vi "Results_Row_Per_Channel.vi"(0 "Analysis_info_cluster":T1={"Colour"=0, "Inst type"=enum."Pitot-static tube", "Inst name"="Manometer voltage", "Symbol"="U", "Code name"="", "Extra Info"="U", "Inst Array"=enum."PWA", "Extra Titles"=[], "Extra Values"=[], "U"=0.0, "u^2"=0.0, "u^3"=0.0, "u^4"=0.0, "Skew_u"=0.0, "Kurt_u"=0.0, "Sd Error in Mean"=0.0, "% u'/U"=0.0, "X"=0.0, "Y"=0.0, "Z"=0.0, "Timescale integral to 25%"=0.0, "Sd Error in Variance"=0.0, "Calib File"=path "", "Calib Constants"=[], "Output Position"=FALSE, "Full Stats"=FALSE, "Av Sampling Rate"=0.0, "Av No of Samples"=0.0, "Total Meas Time (s)"=0.0, "ADAM Ch Name"=""} {"Sd Error in Variance" format="%.2f"; "Skew_u" format="%.2f"; "% u'/U" format="%.2f"; "Sd Error in Mean" format="%.2f"; "Kurt_u" format="%.2f"; "u^4" format="%.2f"; "u^3" format="%.2f"; "U" format="%.2f"; "u^2" format="%.2f"}) -> (1 "Channel Names":string[](array[string]), 2 "Channel Values":string[](array[string]))   [LabVIEW 2015]
uses:
  Controls/Analysis_info_cluster.ctl
  Controls/Inst_type.ctl
  Controls/Instrument_Array.ctl
  Controls/Post_Process.ctl
  Globals/Trav_pos_global.vi
  Acquisition/PWA/PWAtasksGLOBAL.vi
  Globals/Meas_global.vi
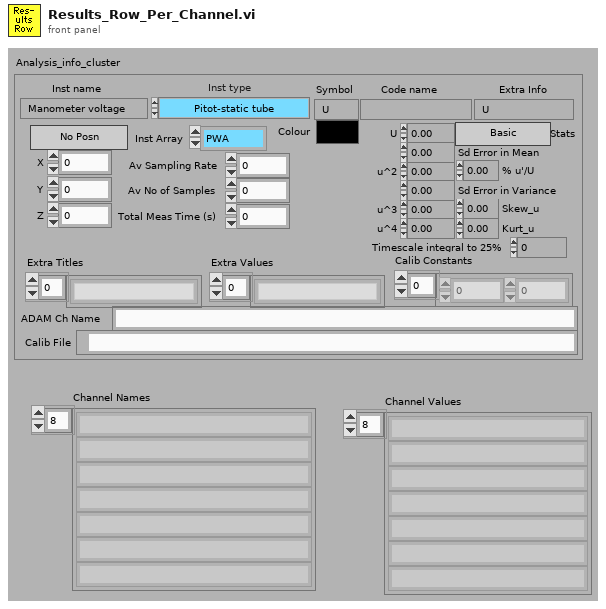
[diagram p1: front panel]
types:
  T1 = typedef "Analysis_info_cluster.ctl" = cluster{"Colour":u32, "Inst type":T2, "Inst name":string, "Symbol":string, "Code name":string, "Extra Info":string, "Inst Array":T3, "Extra Titles":string[], "Extra Values":string[], "U":dbl, "u^2":dbl, "u^3":dbl, "u^4":dbl, "Skew_u":dbl, "Kurt_u":dbl, "Sd Error in Mean":dbl, "% u'/U":dbl, "X":dbl, "Y":dbl, "Z":dbl, "Timescale integral to 25%":dbl, "Sd Error in Variance":dbl, "Calib File":path, "Calib Constants":dbl[], "Output Position":bool, "Full Stats":bool, "Av Sampling Rate":dbl, "Av No of Samples":dbl, "Total Meas Time (s)":dbl, "ADAM Ch Name":string}
  T2 = typedef "Inst_type.ctl" = enum16{"Propeller anemometer", "Raw voltage", "Pressure Transducer", "Pitot-static tube", "Preston tube", "Hot wire", "Cross wire 1", "Cross wire 2", "Generic Linear", "Generic Polynomial", "Generic BackPoly", "Fast FID", "Thermocouple", "Cold wire", "Pulsed Wire", "LDA Vel", "LDA Tran time", "LDA Arr time", "Microphone"}
  T3 = typedef "Instrument_Array.ctl" = enum16{"PWA", "LDA", "Analogue"}
  T4 = enum16{"Mean only", "2nd Order Stats", "4th Order Stats"}
  T5 = typedef "Post_Process.ctl" = enum16{"Take New Data", "Post Process Raw Data File"}
  T6 = typedef "Tunnel_Coordinates.ctl" = enum16{"Work in Tunnel Coordinates", "Work in Model Coordinates"}
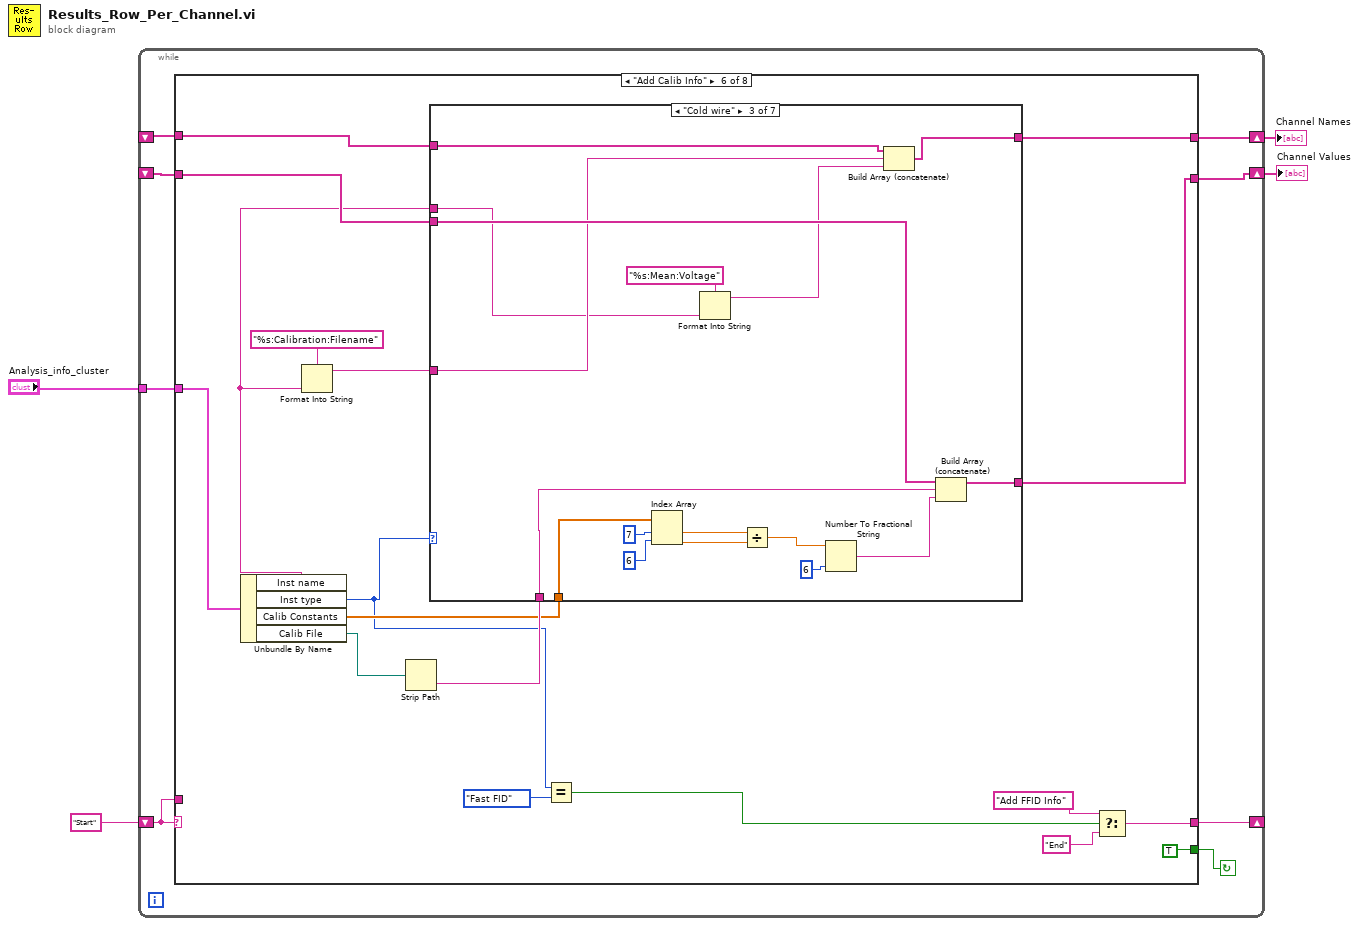
[diagram p0: block diagram]
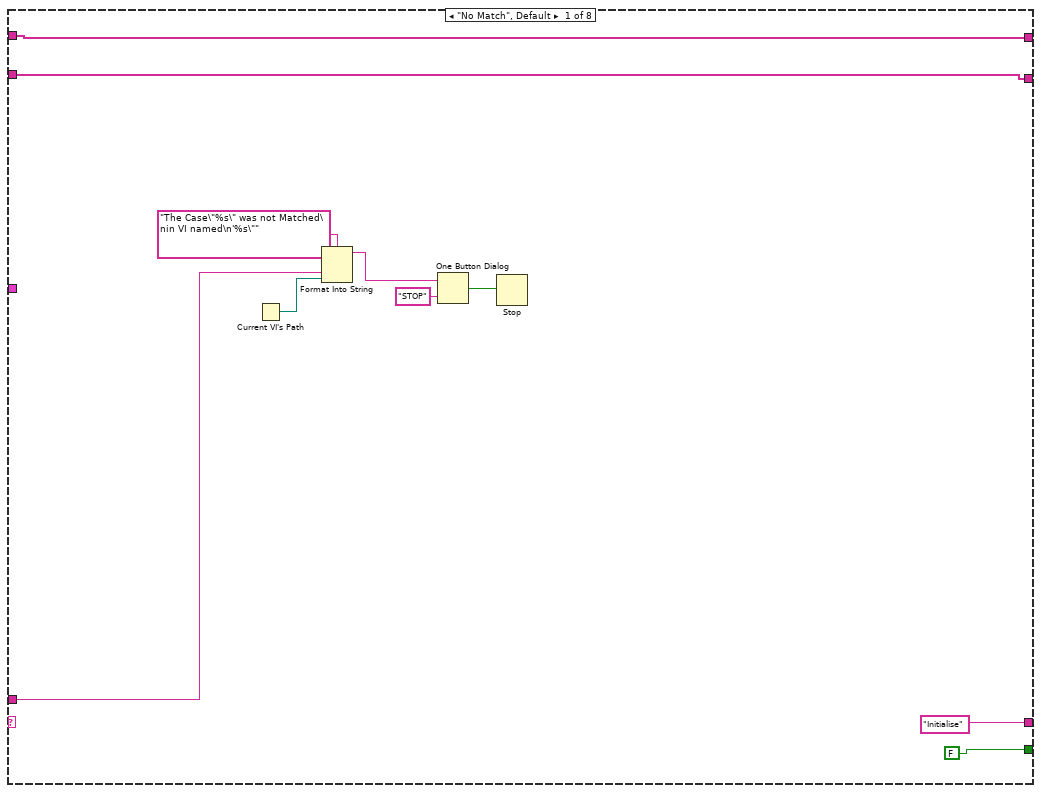
[diagram p2: hidden frame]
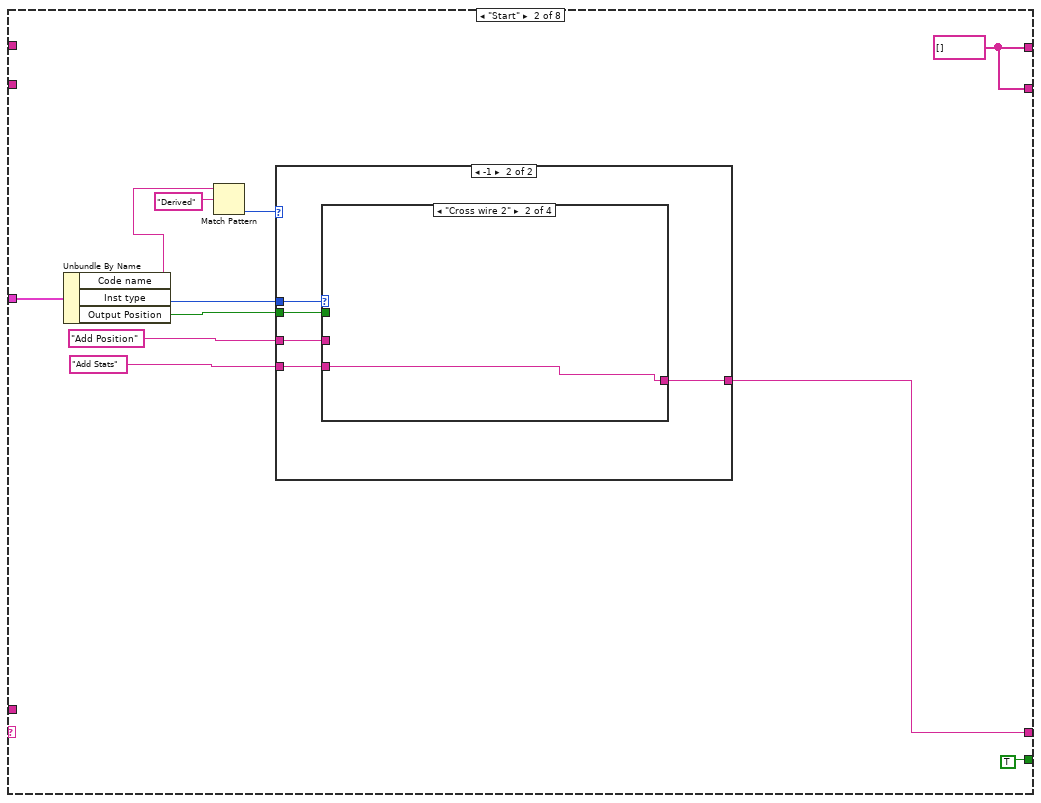
[diagram p3: hidden frame]
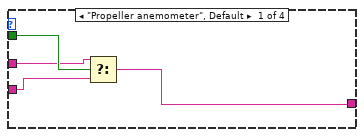
[diagram p5: hidden frame]
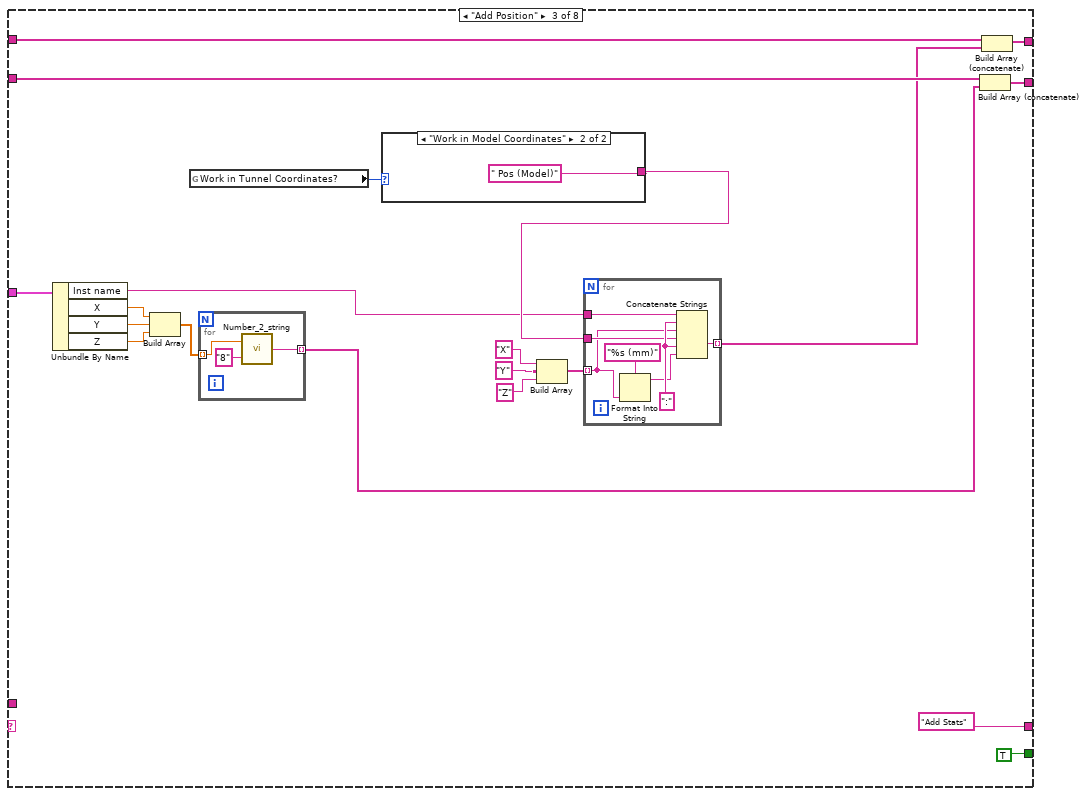
[diagram p8: hidden frame]
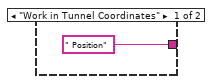
[diagram p9: hidden frame]
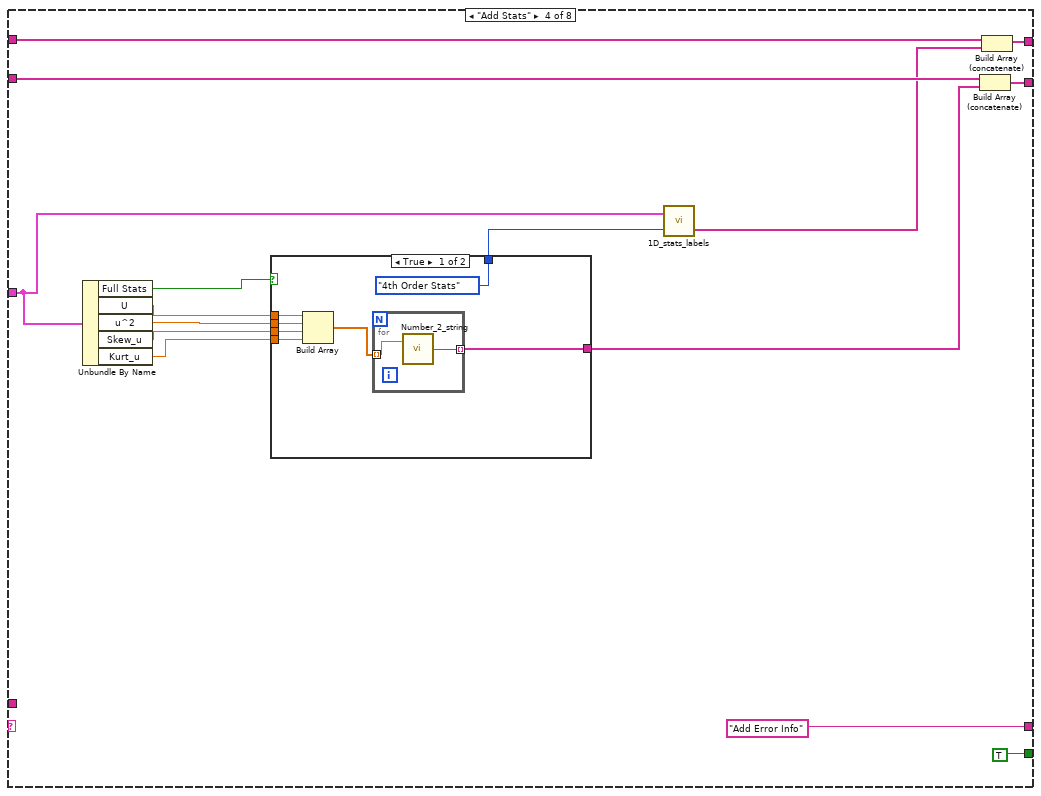
[diagram p10: hidden frame]
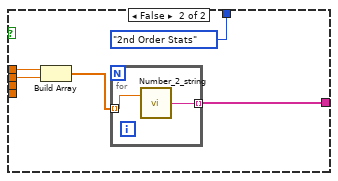
[diagram p11: hidden frame]
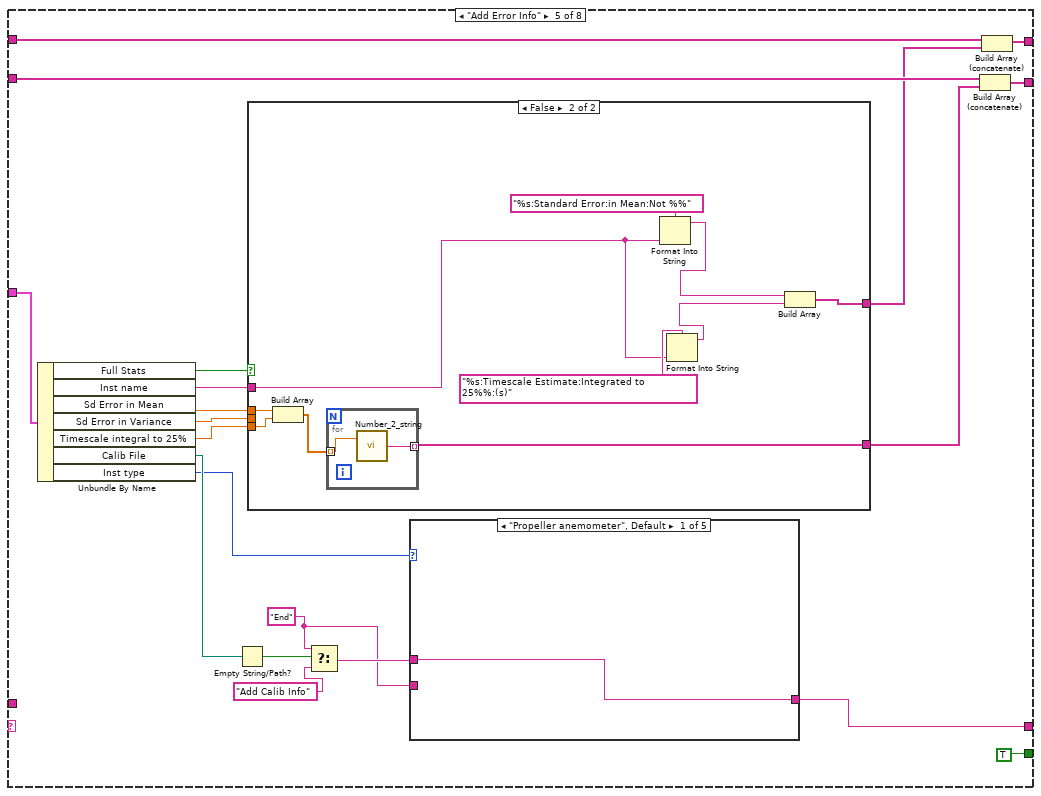
[diagram p12: hidden frame]
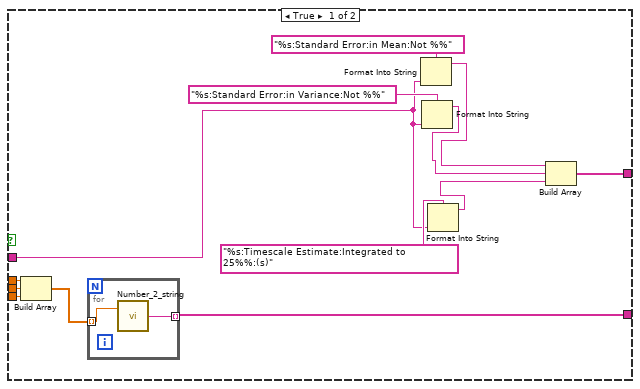
[diagram p13: hidden frame]
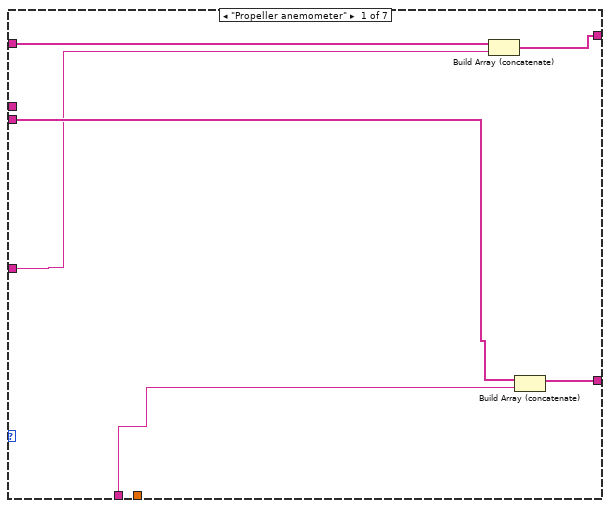
[diagram p18: hidden frame]
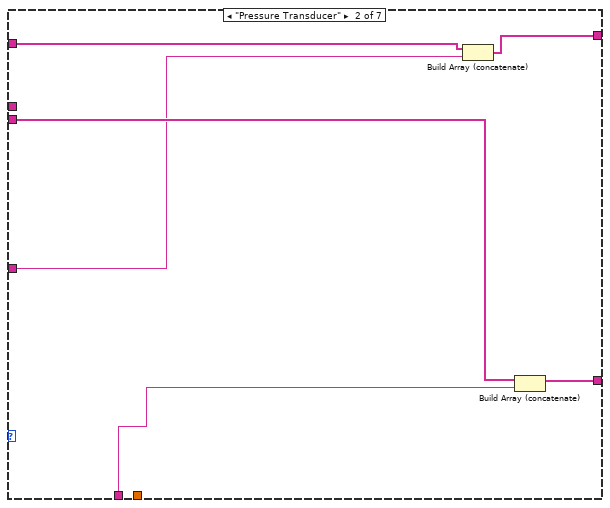
[diagram p19: hidden frame]
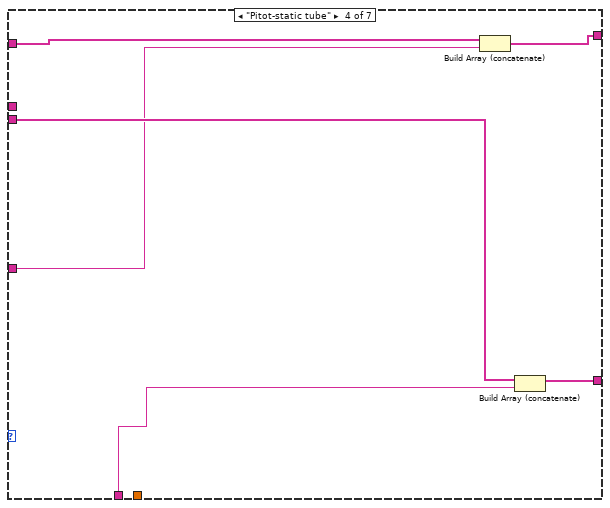
[diagram p20: hidden frame]
diagram:
  n1 = while {
    shift-left: "Start" -> [w10]
    shift-right: [w11] -> _
    shift-right: [w5] -> w1
    shift-left: _ -> [w6]
    shift-right: [w8] -> w2
    shift-left: _ -> [w7]
    tunnel: "Analysis_info_cluster" -> [w9]
    stop <- w12 continue-if-true
    n2 = case shown="\"Add Calib Info\"" w10 {
      tunnel: [FALSE TRUE TRUE TRUE TRUE TRUE TRUE FALSE] -> w12
      tunnel: ["Initialise" w30 "Add Stats" "Add Error Info" w113 w164 "End" "End"] -> w11
      tunnel: w10 -> [w18 _ _ _ _ _ _ _]
      tunnel: w9 -> [_ w32 w58 w84 w122 w178 w277 w298]
      tunnel: [w13 w28 w51 w89 w126 w174 w281 w292] -> w8
      tunnel: w7 -> [w13 _ w50 w88 w125 w176 w280 w295]
      tunnel: w6 -> [w14 _ w49 w87 w124 w171 w279 w297]
      tunnel: [w14 w28 w48 w86 w123 w169 w278 w293] -> w5
      frame "No Match", Default {
        n3 = Current VI's Path() -> (path=w17:path)
        n4 = Format Into String(format string="The Case\"%s\" was not Matched\nin VI named\n'%s\"" ("Format String"), w18, w17) -> (resulting string=w21:string)  [unwired: 2 in, 1 out]
        n5 = One Button Dialog(message=w21, button name ("OK")="STOP") -> (true=w19:bool)
        n6 = Stop(stop? (T)=w19) -> ()
      }
      frame "Start" {
        w28 = string[] []
        n7 = Unbundle By Name(w32) -> ("Code name"=w25:string, "Inst type"=w31:T2, "Output Position"=w23:bool)
        n8 = Match Pattern(string=w25, regular expression="Derived") -> (offset past match=w24:i32)  [unwired: 1 in, 3 out]
        n9 = case shown="-1" w24 {
          tunnel: w31 -> [_ w39]
          tunnel: [w34 w38] -> w30
          tunnel: "Add Position" -> [_ w37]
          tunnel: "Add Stats" -> [w34 w36]
          tunnel: w23 -> [_ w35]
          frame 0, Default {
          }
          frame -1 {
            n10 = case shown="\"Cross wire 2\"" w39 {
              tunnel: [w40 w44 w45 w46] -> w38
              tunnel: w37 -> [w42 _ _ _]
              tunnel: w36 -> [w41 w44 w45 w46]
              tunnel: w35 -> [w43 _ _ _]
              frame "Propeller anemometer", Default {
                n11 = Select(t=w42, s=w43, f=w41) -> (s? t:f=w40:string)
              }
              frame "Cross wire 2" {
              }
              frame "LDA Tran time" {
              }
              frame "LDA Arr time" {
              }
            }
          }
        }
      }
      frame "Add Position" {
        n12 = Unbundle By Name(w58) -> ("Inst name"=w57:string, "X"=w56:dbl, "Y"=w55:dbl, "Z"=w54:dbl)
        n13 = Build Array(w56, w55, w54) -> (w53:dbl[])
        n14 = global read "Trav_pos_global.vi" "Work in Tunnel Coordinates?"() -> (w64:T6)
        n15 = for {
          tunnel: w53 -> [w69] mode=indexing
          tunnel: [w68] -> w52 mode=indexing
          n16 = call "Number_2_string.vi"("precision"="8", "number"=w69) -> ("String"=w68:string)
        }
        n17 = case shown="\"Work in Model Coordinates\"" w64 {
          tunnel: [" Position" " Pos (Model)"] -> w59
          frame "Work in Tunnel Coordinates" {
          }
          frame "Work in Model Coordinates" {
          }
        }
        n18 = Build Array("X", "Y", "Z") -> (w63:string[])
        n19 = for {
          tunnel: w63 -> [w72] mode=indexing
          tunnel: w57 -> [w76]
          tunnel: [w74] -> w47 mode=indexing
          tunnel: w59 -> [w73]
          w75 = ":" ("Substring")
          n20 = Format Into String(format string="%s (mm)", w72) -> (resulting string=w70:string)  [unwired: 2 in, 1 out]
          n21 = Concatenate Strings(w76, w75, w72, w73, w75, w70) -> (w74:string)
        }
        n22 = Build Array (concatenate)(w50, w52) -> (w51:string[])
        n23 = Build Array (concatenate)(w49, w47) -> (w48:string[])
      }
      frame "Add Stats" {
        n24 = Unbundle By Name(w84) -> ("Full Stats"=w80:bool, "U"=w93:dbl, "u^2"=w92:dbl, "Skew_u"=w91:dbl, "Kurt_u"=w85:dbl)
        n25 = case shown="True" w80 {
          tunnel: w93 -> [w100 w107]
          tunnel: w92 -> [w99 w106]
          tunnel: w91 -> [w98 _]
          tunnel: [w96 w104] -> w90
          tunnel: w85 -> [w95 _]
          tunnel: [T4."4th Order Stats" ("Mode selector") T4."2nd Order Stats" ("Mode selector")] -> w81
          frame True {
            n26 = Build Array(w100, w99, w98, w95) -> (w97:dbl[])
            n27 = for {
              tunnel: w97 -> [w102] mode=indexing
              tunnel: [w101] -> w96 mode=indexing
              n28 = call "Number_2_string.vi"("number"=w102) -> ("String"=w101:string)  [unwired: 1 in]
            }
          }
          frame False {
            n29 = Build Array(w107, w106) -> (w105:dbl[])
            n30 = for {
              tunnel: w105 -> [w109] mode=indexing
              tunnel: [w108] -> w104 mode=indexing
              n31 = call "Number_2_string.vi"("number"=w109) -> ("String"=w108:string)  [unwired: 1 in]
            }
          }
        }
        n32 = call "1D_stats_labels.vi"("Mode selector"=w81, "Analysis Info Cluster"=w84) -> ("Output"=w83:string[])  [unwired: 1 in]
        n33 = Build Array (concatenate)(w88, w90) -> (w89:string[])
        n34 = Build Array (concatenate)(w87, w83) -> (w86:string[])
      }
      frame "Add Error Info" {
        w111 = "End"
        n35 = Unbundle By Name(w122) -> ("Full Stats"=w110:bool, "Inst name"=w121:string, "Sd Error in Mean"=w128:dbl, "Sd Error in Variance"=w119:dbl, "Timescale integral to 25%"=w118:dbl, "Calib File"=w117:path, "Inst type"=w112:T2)
        n36 = Empty String/Path?(string/path=w117) -> (empty?=w116:bool)
        n37 = case shown="False" w110 {
          tunnel: w128 -> [w142 w154]
          tunnel: [w140 w152] -> w127
          tunnel: w121 -> [w133 w147]
          tunnel: [w132 w146] -> w120
          tunnel: w119 -> [w131 _]
          tunnel: w118 -> [w130 w145]
          frame True {
            n38 = Build Array(w142, w131, w130) -> (w141:dbl[])
            n39 = for {
              tunnel: w141 -> [w144] mode=indexing
              tunnel: [w143] -> w140 mode=indexing
              n40 = call "Number_2_string.vi"("number"=w144) -> ("String"=w143:string)  [unwired: 1 in]
            }
            n41 = Format Into String(format string="%s:Standard Error:in Mean:Not %%", w133) -> (resulting string=w135:string)  [unwired: 2 in, 1 out]
            n42 = Format Into String(format string="%s:Standard Error:in Variance:Not %%", w133) -> (resulting string=w137:string)  [unwired: 2 in, 1 out]
            n43 = Format Into String(format string="%s:Timescale Estimate:Integrated to 25%%:(s)", w133) -> (resulting string=w139:string)  [unwired: 2 in, 1 out]
            n44 = Build Array(w135, w137, w139) -> (w132:string[])
          }
          frame False {
            n45 = Build Array(w154, w145) -> (w153:dbl[])
            n46 = for {
              tunnel: w153 -> [w156] mode=indexing
              tunnel: [w155] -> w152 mode=indexing
              n47 = call "Number_2_string.vi"("number"=w156) -> ("String"=w155:string)  [unwired: 1 in]
            }
            n48 = Format Into String(format string="%s:Standard Error:in Mean:Not %%", w147) -> (resulting string=w149:string)  [unwired: 2 in, 1 out]
            n49 = Format Into String(format string="%s:Timescale Estimate:Integrated to 25%%:(s)", w147) -> (resulting string=w151:string)  [unwired: 2 in, 1 out]
            n50 = Build Array(w149, w151) -> (w146:string[])
          }
        }
        n51 = Select(t=w111, s=w116, f="Add Calib Info") -> (s? t:f=w114:string)
        n52 = case shown="\"Propeller anemometer\", Default" w112 {
          tunnel: [w157 w158 w159 w160 w161] -> w113
          tunnel: w114 -> [w157 _ _ _ _]
          tunnel: w111 -> [_ w158 w159 w160 w161]
          frame "Propeller anemometer", Default {
          }
          frame "Cross wire 2" {
          }
          frame "LDA Tran time" {
          }
          frame "LDA Arr time" {
          }
          frame "Raw voltage" {
          }
        }
        n53 = Build Array (concatenate)(w125, w127) -> (w126:string[])
        n54 = Build Array (concatenate)(w124, w120) -> (w123:string[])
      }
      frame "Add Calib Info" {
        n55 = Unbundle By Name(w178) -> ("Inst name"=w168:string, "Inst type"=w167:T2, "Calib Constants"=w173:dbl[], "Calib File"=w177:path)
        n56 = Format Into String(format string="%s:Calibration:Filename" ("Format String"), w168) -> (resulting string=w170:string)  [unwired: 2 in, 1 out]
        n57 = Strip Path(path=w177) -> (name=w175:string)  [unwired: 1 out]
        n58 = case shown="\"Cold wire\"" w167 {
          tunnel: [w185 w190 w207 w213 w219 w226 w249] -> w174
          tunnel: w176 -> [w183 w191 w208 w214 w220 w227 w250]
          tunnel: w175 -> [w184 w189 w206 w212 w218 _ w243]
          tunnel: w173 -> [_ _ w199 _ _ _ w242]
          tunnel: w171 -> [w182 w188 w205 w211 w217 w223 w235]
          tunnel: w170 -> [w180 w187 w204 w209 w216 w221 w234]
          tunnel: [w181 w186 w203 w210 w215 w222 w229] -> w169
          tunnel: w168 -> [_ _ w201 _ _ _ w228]
          frame "Propeller anemometer" {
            n59 = Build Array (concatenate)(w182, w180) -> (w181:string[])
            n60 = Build Array (concatenate)(w183, w184) -> (w185:string[])
          }
          frame "Pressure Transducer" {
            n61 = Build Array (concatenate)(w188, w187) -> (w186:string[])
            n62 = Build Array (concatenate)(w191, w189) -> (w190:string[])
          }
          frame "Cold wire" {
            n63 = Index Array(array=w199, index #1=7 ("index"), index #2=6 ("index")) -> (element #1=w193:dbl, element #2=w192:dbl)
            n64 = Format Into String(format string="%s:Mean:Voltage" ("Format String"), w201) -> (resulting string=w200:string)  [unwired: 2 in, 1 out]
            n65 = Divide(x=w193, y=w192) -> (x/y=w197:dbl)
            n66 = Number To Fractional String(number=w197, precision (6)=i16 6) -> (F-format string=w195:string)  [unwired: 2 in]
            n67 = Build Array (concatenate)(w205, w204, w200) -> (w203:string[])
            n68 = Build Array (concatenate)(w208, w206, w195) -> (w207:string[])
          }
          frame "Pitot-static tube" {
            n69 = Build Array (concatenate)(w211, w209) -> (w210:string[])
            n70 = Build Array (concatenate)(w214, w212) -> (w213:string[])
          }
          frame "Preston tube" {
            n71 = Build Array (concatenate)(w220, w218) -> (w219:string[])
            n72 = Build Array (concatenate)(w217, w216) -> (w215:string[])
          }
          frame "Pulsed Wire" {
            n73 = global read "PWAtasksGLOBAL.vi" "PWA Calib. File Path"() -> (w225:path)
            n74 = Strip Path(path=w225) -> (name=w224:string)  [unwired: 1 out]
            n75 = Build Array (concatenate)(w223, w221) -> (w222:string[])
            n76 = Build Array (concatenate)(w227, w224) -> (w226:string[])
          }
          frame "Generic Linear", Default {
            n77 = global read "Meas_global.vi" "Post Process"() -> (w245:T5)
            n78 = Index Array(array=w242, index=18 ("Index")) -> (element=w248:dbl)
            n79 = Format Into String(format string="%s:Calibration:Drift:%%" ("Format String"), w228) -> (resulting string=w231:string)  [unwired: 2 in, 1 out]
            n80 = Not A Number/Path/Refnum?(number/path/refnum=w248) -> (NaN/Path/Refnum?=w247:bool)
            n81 = Equal?(x=w245, y=Post_Process."Post Process Raw Data File" ("Post Process")) -> (x = y?=w238:bool)
            n82 = case shown="False" w247 {
              tunnel: [w260 w265] -> w244
              tunnel: w248 -> [w261 _]
              tunnel: w238 -> [_ w267]
              tunnel: w243 -> [_ w264]
              frame False {
                n83 = Number To Fractional String(number=w261, precision (6)=i16 2) -> (F-format string=w260:string)  [unwired: 2 out]
              }
              frame True {
                n84 = Concatenate Strings(w264, "_Drift_Place_Holder" ("Substring")) -> (w266:string)
                n85 = Select(t="No Info", s=w267, f=w266) -> (s? t:f=w265:string)
              }
            }
            n86 = Index Array(array=w242, index=19 ("Index")) -> (element=w241:dbl)
            n87 = Not A Number/Path/Refnum?(number/path/refnum=w241) -> (NaN/Path/Refnum?=w240:bool)
            n88 = case shown="False" w240 {
              tunnel: [w251 w256] -> w239
              tunnel: w241 -> [w252 _]
              tunnel: w238 -> [_ w258]
              tunnel: w243 -> [_ w255]
              frame False {
                n89 = Number To Fractional String(number=w252, precision (6)=i16 2) -> (F-format string=w251:string)  [unwired: 2 out]
              }
              frame True {
                n90 = Concatenate Strings(w255, "_Interval_Place_Holder" ("Substring")) -> (w257:string)
                n91 = Select(t="No Info", s=w258, f=w257) -> (s? t:f=w256:string)
              }
            }
            n92 = Format Into String(format string="%s:Calibration:Interval:Minutes" ("Format String"), w228) -> (resulting string=w230:string)  [unwired: 2 in, 1 out]
            n93 = Build Array (concatenate)(w250, w243, w244, w239) -> (w249:string[])
            n94 = Build Array (concatenate)(w235, w234, w231, w230) -> (w229:string[])
          }
        }
        n95 = Equal?(x=w167, y=Inst_type."Fast FID" ("Inst type")) -> (x = y?=w166:bool)
        n96 = Select(t="Add FFID Info", s=w166, f="End") -> (s? t:f=w164:string)
      }
      frame "Add FFID Info" {
        n97 = Unbundle By Name(w277) -> ("Inst name"=w272:string, "Calib Constants"=w275:dbl[])
        n98 = for {
          tunnel: w275 -> [w291]
          tunnel: i32[] [12, 3, 4, 11, 7] ("Calib Constants") -> [w290] mode=indexing
          tunnel: [w288] -> w273 mode=indexing
          n99 = Index Array(array=w291, index=w290) -> (element=w289:dbl)
          n100 = call "Number_2_string.vi"("number"=w289) -> ("String"=w288:string)  [unwired: 1 in]
        }
        n101 = for {
          tunnel: string[] ["Intermittency", "Bkgnd", "Bkgnd Variance", "Threshold", "Calibration"] ("appended array") -> [w284] mode=indexing
          tunnel: w272 -> [w285]
          tunnel: [w286] -> w271 mode=indexing
          tunnel: string[] ["", "ppm", "ppm^2", "ppm", "ppm/%Density"] ("appended array") -> [w283] mode=indexing
          w287 = ":" ("Substring")
          n102 = Concatenate Strings(w285, w287, w284, w287, w283) -> (w286:string)
        }
        n103 = Build Array (concatenate)(w280, w273) -> (w281:string[])
        n104 = Build Array (concatenate)(w279, w271) -> (w278:string[])
      }
      frame "End" {
        n105 = Unbundle By Name(w298) -> ("Extra Titles"=w296:string[], "Extra Values"=w294:string[])
        n106 = Build Array (concatenate)(w297, w296) -> (w293:string[])
        n107 = Build Array (concatenate)(w295, w294) -> (w292:string[])
      }
    }
  }
  "Channel Names" <- w1
  "Channel Values" <- w2
